vi "Update display contrast.vi"(8 "error in (no error)":errorcluster, 11 "DAQOrcaFlash in":refnum<class "DAQOrcaFlash.lvclass">) -> (0 "error out":errorcluster, 3 "DAQOrcaFlash out":refnum<class "DAQOrcaFlash.lvclass">)   [LabVIEW 2012, in "DAQOrcaFlash.lvclass"]
uses:
  DAQOrcaFlash.lvclass
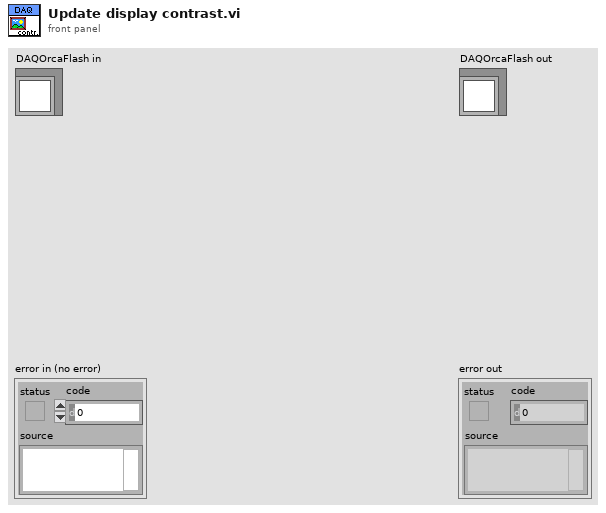
[diagram p1: front panel]
types:
  T1 = cluster{"Conversion Method":u32, "Minimum Value":i32, "Maximum Value":i32, "# Shifts":i32}
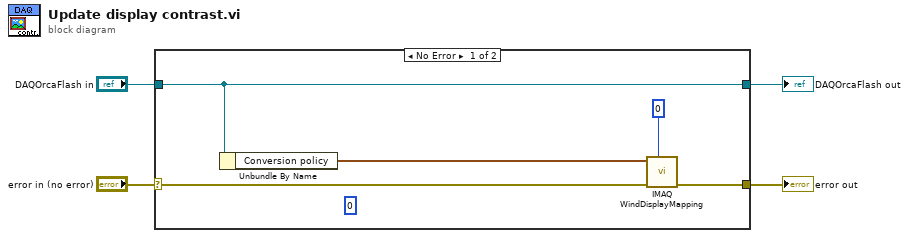
[diagram p0: block diagram]
diagram:
  n1 = case shown="No Error" "error in (no error)" {
    selector: "error in (no error)" -> [w7 w11]
    tunnel: [w6 w11] -> w3
    tunnel: [w9 w10] -> w1
    tunnel: "DAQOrcaFlash in" -> [w9 w10]
    frame No Error {
      (unwired) u32 0 ("Conversion Method")
      n2 = Unbundle By Name(w9) -> ("Conversion policy"=w5:T1)
      n3 = call "IMAQ WindDisplayMapping"("Window Number (0...15)"=0, "error in (no error)"=w7, "Conversion Policy (Default)"=w5) -> ("error out"=w6:errorcluster)  [unwired: 7 in, 1 out]
    }
    frame Error {
    }
  }
  "error out" <- w3
  "DAQOrcaFlash out" <- w1
